vi "Graph data.vi"(8 "error in (no error)":errorcluster, 10 "signal out":waveform(dbl), 11 "GUI Actor in":refnum<class "GUI Actor.lvclass">) -> (0 "error out":errorcluster, 3 "GUI Actor out":refnum<class "GUI Actor.lvclass">)   [LabVIEW 2019, in "GUI Actor.lvlib" / "GUI Actor.lvclass"]
uses:
  GUI Actor.lvclass
  GUI Actor.lvclass/GUI Actor.ctl
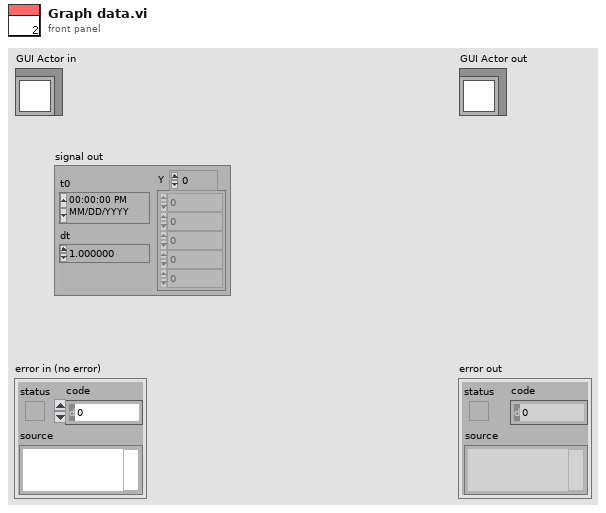
[diagram p1: front panel]
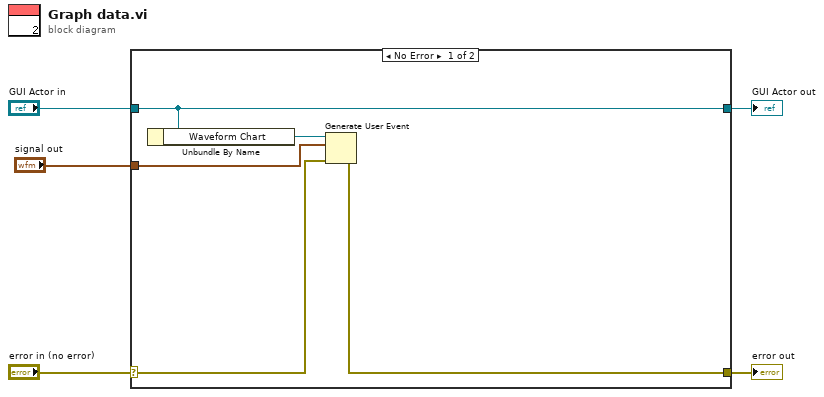
[diagram p0: block diagram]
diagram:
  n1 = case shown="No Error" "error in (no error)" {
    selector: "error in (no error)" -> [w8 w12]
    tunnel: [w7 w12] -> w4
    tunnel: [w10 w11] -> w2
    tunnel: "GUI Actor in" -> [w10 w11]
    tunnel: "signal out" -> [w6 _]
    frame No Error {
      n2 = Unbundle By Name(w10) -> ("Waveform Chart"=w9:refnum<user-event>)
      n3 = Generate User Event(user event=w9, event data cluster=w6, error in=w8) -> (error out=w7:errorcluster)  [unwired: 1 in, 1 out]
    }
    frame Error {
    }
  }
  "error out" <- w4
  "GUI Actor out" <- w2
